vi "RawStringtoCluster.vi"(8 "error in (no error)":errorcluster, 11 "Raw String":string) -> (0 "error out":errorcluster, 3 "DataIn":T1)   [LabVIEW 2017]
doc: "This VI converts the JSON string read in from the UDP connection into a cluster."
uses:
  TypeDefs/dataIn.ctl
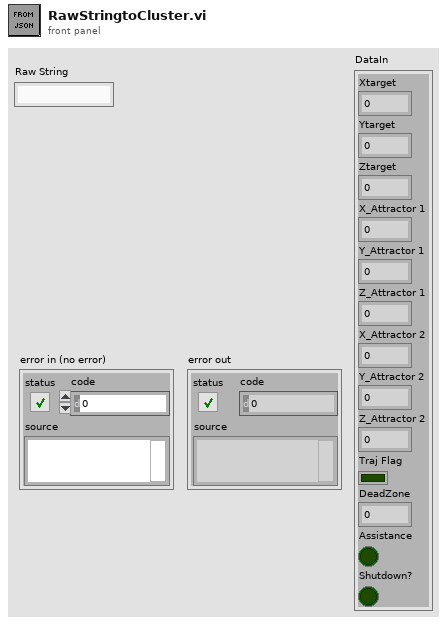
[diagram p1: front panel]
types:
  T1 = typedef "dataIn.ctl" = cluster{"Xtarget":dbl, "Ytarget":dbl, "Ztarget":dbl, "X_Attractor 1":dbl, "Y_Attractor 1":dbl, "Z_Attractor 1":dbl, "X_Attractor 2":dbl, "Y_Attractor 2":dbl, "Z_Attractor 2":dbl, "Traj Flag":bool, "DeadZone":dbl, "Assistance":bool, "Shutdown?":bool}
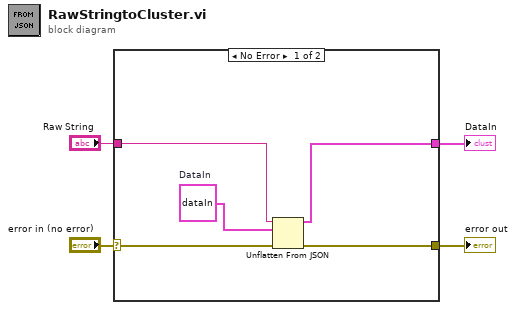
[diagram p0: block diagram]
diagram:
  n1 = case shown="No Error" "error in (no error)" {
    selector: "error in (no error)" -> [w9 w10]
    tunnel: "Raw String" -> [w7 _]
    tunnel: [w8 w10] -> w2
    tunnel: [w5 _] -> w1
    frame No Error {
      w6 = T1 {"Xtarget"=0.0, "Ytarget"=0.0, "Ztarget"=0.0, "X_Attractor 1"=0.0, "Y_Attractor 1"=0.0, "Z_Attractor 1"=0.0, "X_Attractor 2"=0.0, "Y_Attractor 2"=0.0, "Z_Attractor 2"=0.0, "Traj Flag"=FALSE, "DeadZone"=0.0, "Assistance"=FALSE, "Shutdown?"=FALSE}  # DataIn
      n2 = Unflatten From JSON(JSON string=w7, type and defaults=w6, error in (no error)=w9) -> (value=w5:T1, error out=w8:errorcluster)  [unwired: 4 in]
    }
    frame Error {
    }
  }
  "error out" <- w2
  "DataIn" <- w1
